vi "json_Get_AddTopic.vi"(8 "error in":errorcluster, 11 "ReadCMD_0":string="{\"ID\": \"b9b762fb-e465-4f6a-bde5-995dda67237b\", \"TO\": \"845CF3525B43\", \"FROM\": \"C87F542F1180\", \"CMD\": 0, \"CONTENT\": [{\"HOSTNAME\": \"SI-AGT01\", \"MAC\": \"845CF3525B43\", \"IP\": \"172.20.10.10\", \"CENTER_NAME\": \"C87F542F1180\", \"ADD_TOPIC\": \"topic/PC/845CF3525B43\", \"REQ_ID\": \"38A46EA6-1EA1-4C1D-82A7-A29BD9BCAD25\"}], \"STATUS\": true, \"ERRCODE\": \"\", \"ERRMSG\": \"\", \"TIMESTAMP\": 1759035794") -> (0 "error out":errorcluster, 3 "AddTopic":string)   [LabVIEW 2020]
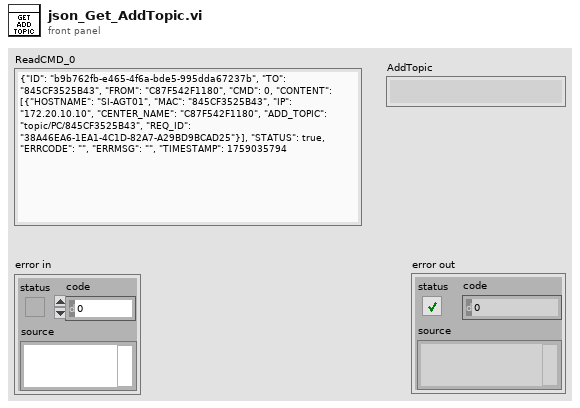
[diagram p1: front panel]
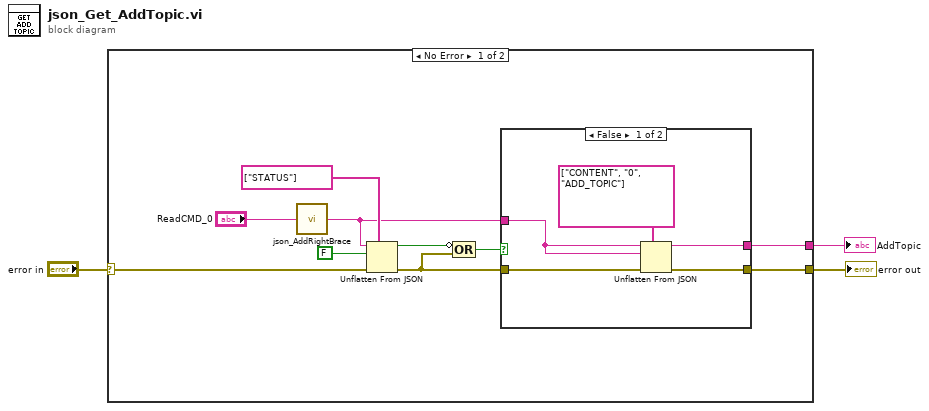
[diagram p0: block diagram]
diagram:
  n1 = case shown="No Error" "error in" {
    selector: "error in" -> [w4 w19]
    tunnel: [w7 w19] -> w3
    tunnel: [w6 _] -> w2
    frame No Error {
      n2 = call "json_AddRightBrace.vi"("ReadCMD_0"="ReadCMD_0") -> ("+}"=w5:string)
      n3 = Unflatten From JSON(path=string[] ["STATUS"], JSON string=w5, type and defaults=FALSE, error in (no error)=w4) -> (value=w11:bool, error out=w10:errorcluster)  [unwired: 3 in]
      n4 = Compound Arithmetic op=OR(invert w11, w10) -> (w8:bool)
      n5 = case shown="False" w8 {
        tunnel: w10 -> [w17 _]
        tunnel: w5 -> [w16 _]
        tunnel: [w15 _] -> w7
        tunnel: [w14 _] -> w6
        frame False {
          n6 = Unflatten From JSON(path=string[] ["CONTENT", "0", "ADD_TOPIC"], JSON string=w16, type and defaults=w16, error in (no error)=w17) -> (value=w14:string, error out=w15:errorcluster)  [unwired: 3 in]
        }
        frame True {
        }
      }
    }
    frame Error {
    }
  }
  "error out" <- w3
  "AddTopic" <- w2
